vi "Pos2ndStrikerAfterPass.vi"(9 "AI Parameters":T1={"GotoKick"={"Dist do cone a frente"=150.0, "attacker farback"=1500.0, "Perto"=300.0, "min dist to kick"=150.0, "kick eps"=0.0, "Time to transition"=0.05}, "Attacker"={"CC chute"=0.09, "CC passe"=0.045, "Kick Force"=100.0, "ball-robot Kick"=200.0, "ball-robot Pass"=0.3, "drible\nAttk"=FALSE}, "Defender"={"D max"=1700.0, "Vel p/ robô av"=1000.0, "Kick Force"=100.0, "D atk-def"=0.0, "D farback"=0.0, "drible\ndef"=FALSE, "drible\ngoalie"=FALSE}, "Timeout"={"Field/v in x"=6.0, "Dist Robots"=300, "Dist up in y"=300}, "Pose Striker"={"dist"=200.0, "Numeric"=-4.0, "dist 2"=200.0, "drible\nstriker"=FALSE}, "Dist Stop"=300.0, "D ball out"=200, "D central gap "=150.0, "T pass"=0.0, "Force ++"=0.0, "range kick"=0.0, "Chute alto"=TRUE, "Marcador novo"=TRUE, "drible"=FALSE, "D drible"=300.0, "Versão Striker"=enum."3", "Defesa"=enum."ManMark", "Marcador"=enum."Marcar Segundo mais perigoso", "Receptor passe"=enum."2nd Striker", "Área"=enum."Quadrada"} {"D drible" format="%#_13g"; "D central gap" format="%#_13g"; "Dist Stop" format="%#_13g"; "Pose Striker"."Numeric" format="%#_13g"; "Defender"."Kick Force" format="%#_13g"; "Defender"."Vel p/ robô av" format="%#_13g"; "Attacker"."ball-robot Kick" format="%#_13g"; "Attacker"."Kick Force" format="%#_13g"; "Attacker"."CC passe" format="%#_13g"; "Attacker"."CC chute" format="%#_13g"; "GotoKick"."kick eps" format="%#_13g"; "GotoKick"."min dist to kick" format="%#_13g"; "GotoKick"."Perto" format="%#_13g"; "GotoKick"."attacker farback" format="%#_13g"; "GotoKick"."Dist do cone a frente" format="%#_13g"}, 10 "IA Input":T2={"our_robots"=[], "enemy_robots"=[], "balls"=[], "geometry"={"line_width"=0, "field_length"=0, "field_width"=0, "boundary_width"=0, "referee_width"=0, "goal_width"=0, "goal_depth"=0, "goal_wall_width"=0, "center_circle_radius"=0, "defense_radius"=0, "defense_stretch"=0, "free_kick_from_defense_dist"=0, "penalty_spot_from_field_line_dist"=0, "penalty_line_from_spot_dist"=0}, "IA Judge"={"stage"="", "command"="", "our_goalie_id"=0.0, "enemy_goalie_id"=0.0, "command enum"=enum."Halt", "Time"=enum."Azul"}, "Received Timestamp"=timestamp(0 s since 1904-01-01), "Events"={"Touch"=FALSE, "Ball out"=FALSE, "id touch"=0.0, "Ball out of \nVision"=FALSE, "Ball inside \nGoalie area"=FALSE, "Robot not responding"=FALSE, "Robots responding status"=[1.0, 1.0, 1.0, 1.0, 1.0, 1.0], "Enemy Ball \nPossession"=FALSE, "Pass State"=FALSE, "id end of pass"=0.0, "Kick"=FALSE, "Id ini Possession"=0.0, "Ball Possesion"=FALSE, "Id Possesion"=0.0, "Direct Kick"=FALSE, "2nd Strk Ativo"=FALSE}}, 11 "Robot in":T3={"id"=5, "function"=enum."Attacker", "x"=-1842.5054931640625, "y"=520.60986328125, "orientation"=-2.7555055618286133, "v_tangent"=0.0, "v_normal"=0.0, "v_ang"=0.0, "kick_x"=0.0, "kick_z"=0.0, "dribble"=FALSE, "Timestamp"=timestamp(2082758857.4639893 s since 1904-01-01), "estimatives"={"est_v_tangent"=0.0, "est_v_normal"=0.0, "est_vx"=0.0, "est_vy"=0.0, "Pos Robot Est"=[]}, "dest_x_kick"=0.0, "dest_y_kick"=0.0, "Gap Coord"=[], "States"=enum."GoToTangent", "Path "=[], "Path  Smooth"=[], "Dest"=[]}) -> (3 "Robot out":T3={"id"=5, "function"=enum."Attacker", "x"=-1842.5054931640625, "y"=520.60986328125, "orientation"=-2.7555055618286133, "v_tangent"=-0.08361641967936218, "v_normal"=-0.20513016702014014, "v_ang"=0.24456003022714357, "kick_x"=0.0, "kick_z"=0.0, "dribble"=FALSE, "Timestamp"=timestamp(2082758857.4639893 s since 1904-01-01), "estimatives"={"est_v_tangent"=0.0, "est_v_normal"=0.0, "est_vx"=0.0, "est_vy"=0.0, "Pos Robot Est"=[]}, "dest_x_kick"=0.0, "dest_y_kick"=0.0, "Gap Coord"=[], "States"=enum."GoToTangent", "Path "=[], "Path  Smooth"=[], "Dest"=[]})   [LabVIEW 2017]
uses:
  Core/AI Robot.ctl
  Functions Enum.ctl
  AttackerStates.ctl
  Path Planning/RRT/PathDests.ctl
  Path Planning/RRT/PathDest.ctl
  Core/AI Input.ctl
  Core/AI Ball.ctl
  Core/Field Size.ctl
  Core/AI Judge.ctl
  Command Enum.ctl
  Util/Events/Events.ctl
  AI Parameters.ctl
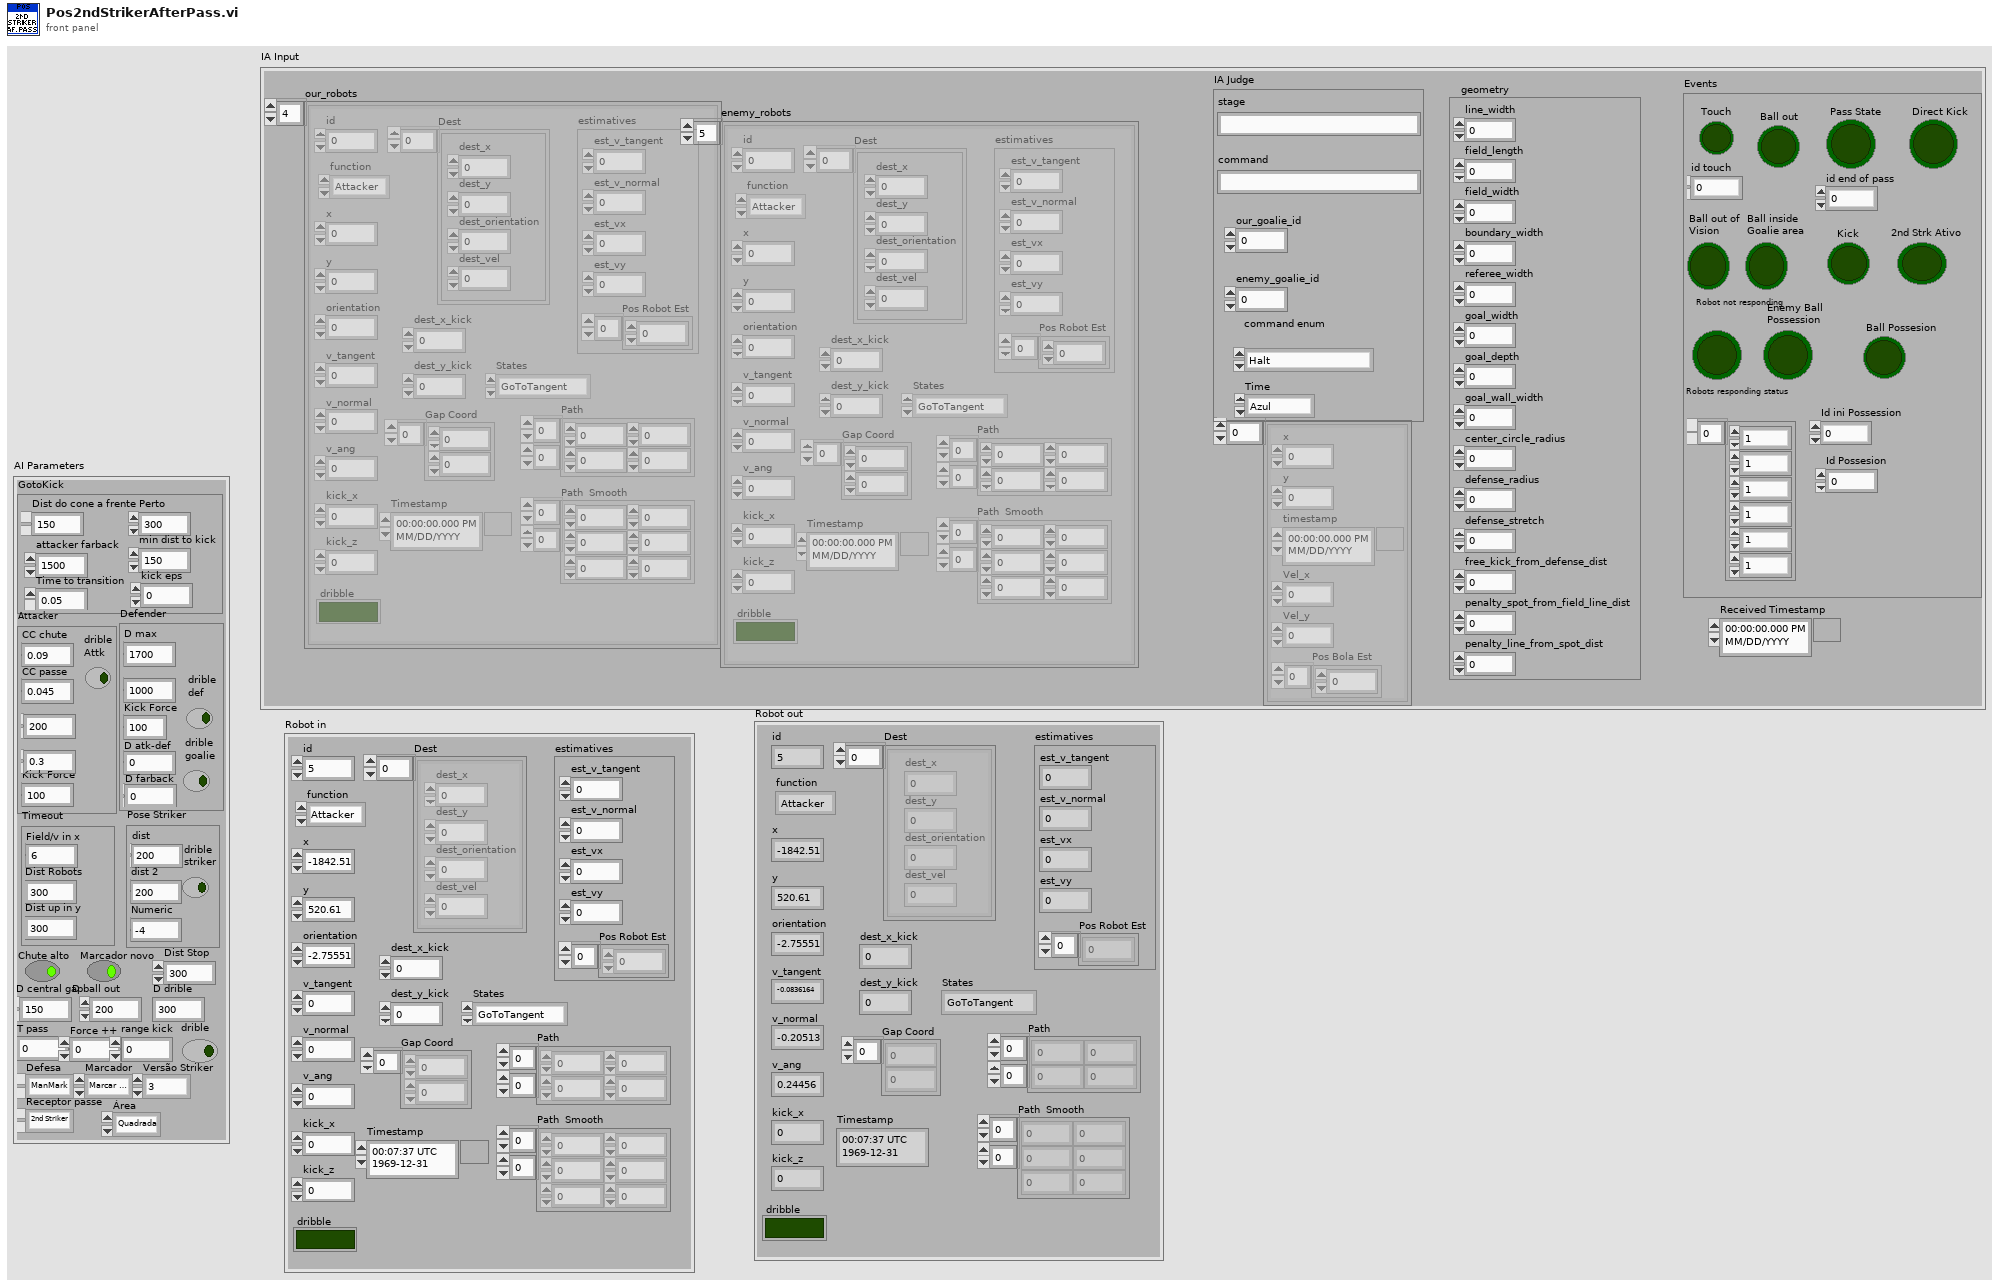
[diagram p1: front panel]
types:
  T1 = typedef "AI Parameters.ctl" = cluster{"GotoKick":cluster{"Dist do cone a frente":dbl, "attacker farback":dbl, "Perto":dbl, "min dist to kick":dbl, "kick eps":dbl, "Time to transition":dbl}, "Attacker":cluster{"CC chute":dbl, "CC passe":dbl, "Kick Force":dbl, "ball-robot Kick":dbl, "ball-robot Pass":dbl, "drible\nAttk":bool}, "Defender":cluster{"D max":dbl, "Vel p/ robô av":dbl, "Kick Force":dbl, "D atk-def":dbl, "D farback":dbl, "drible\ndef":bool, "drible\ngoalie":bool}, "Timeout":cluster{"Field/v in x":dbl, "Dist Robots":u32, "Dist up in y":u32}, "Pose Striker":cluster{"dist":dbl, "Numeric":dbl, "dist 2":dbl, "drible\nstriker":bool}, "Dist Stop":dbl, "D ball out":i32, "D central gap ":dbl, "T pass":dbl, "Force ++":dbl, "range kick":dbl, "Chute alto":bool, "Marcador novo":bool, "drible":bool, "D drible":dbl, "Versão Striker":enum16{"Auto", "3", "2", "1"}, "Defesa":enum16{"ManMark", "Barreira"}, "Marcador":enum16{"Marcar Segundo mais perigoso", "Marcar o mais perigoso"}, "Receptor passe":enum16{"Auto", "2nd Striker", "Striker"}, "Área":enum16{"Quadrada", "Circular"}}
  T2 = typedef "AI Input.ctl" = cluster{"our_robots":T3[], "enemy_robots":T3[], "balls":T8[], "geometry":T9, "IA Judge":T10, "Received Timestamp":timestamp, "Events":T12}
  T3 = typedef "AI Robot.ctl" = cluster{"id":u32, "function":T4, "x":dbl, "y":dbl, "orientation":dbl, "v_tangent":dbl, "v_normal":dbl, "v_ang":dbl, "kick_x":dbl, "kick_z":dbl, "dribble":bool, "Timestamp":timestamp, "estimatives":cluster{"est_v_tangent":dbl, "est_v_normal":dbl, "est_vx":dbl, "est_vy":dbl, "Pos Robot Est":dbl[]}, "dest_x_kick":dbl, "dest_y_kick":dbl, "Gap Coord":dbl[], "States":T5, "Path ":dbl[][], "Path  Smooth":dbl[][], "Dest":T6}
  T4 = typedef "Functions Enum.ctl" = enum16{"2nd Striker", "Attacker", "Goalie", "Defender", "Striker", "Goto 0", "Dummy", "Kicker", "ZigZag 0", "ZigZag 1", "ZigZag 2", "ZigZag 3", "ZigZag 4", "ZigZag 5", "ZigZag 6", "ZigZag 7", "ZigZag 8", ""}
  T5 = typedef "AttackerStates.ctl" = enum16{"Pass", "GoToTangent", "BallGetting", "GoToKick", ""}
  T6 = typedef "PathDests.ctl" = T7[]
  T7 = typedef "PathDest.ctl" = cluster{"dest_x":dbl, "dest_y":dbl, "dest_orientation":dbl, "dest_vel":dbl}
  T8 = typedef "AI Ball.ctl" = cluster{"x":dbl, "y":dbl, "timestamp":timestamp, "Vel_x":dbl, "Vel_y":dbl, "Pos Bola Est":dbl[]}
  T9 = typedef "Field Size.ctl" = cluster{"line_width":u32, "field_length":u32, "field_width":u32, "boundary_width":u32, "referee_width":u32, "goal_width":u32, "goal_depth":u32, "goal_wall_width":u32, "center_circle_radius":u32, "defense_radius":u32, "defense_stretch":u32, "free_kick_from_defense_dist":u32, "penalty_spot_from_field_line_dist":u32, "penalty_line_from_spot_dist":u32}
  T10 = typedef "AI Judge.ctl" = cluster{"stage":string, "command":string, "our_goalie_id":dbl, "enemy_goalie_id":dbl, "command enum":T11, "Time":enum16{"Azul", "Amarelo"}}
  T11 = typedef "Command Enum.ctl" = enum16{"Halt", "Stop", "Force Start", "PKA Normal Start", "Prepare Kickoff Ally", "PKE Normal Start", "Prepare Kickoff Enemy", "Prepare Penalty Ally", "PPA Normal Start", "Prepare Penalty Enemy", "PPE Normal Start", "Direct Free Enemy", "Direct Free Ally", "Indirect Free Enemy", "Indirect Free Ally", "Timeout Enemy", "Timeout Ally", "Goal Enemy", "Goal Ally", "Ball Placement Enemy", "Ball Placement Ally", "Normal Half Time", "Extra Time Break", "Extra Half Time", "None", "Post Game"}
  T12 = typedef "Events.ctl" = cluster{"Touch":bool, "Ball out":bool, "id touch":dbl, "Ball out of \nVision":bool, "Ball inside \nGoalie area":bool, "Robot not responding":bool, "Robots responding status":dbl[], "Enemy Ball \nPossession":bool, "Pass State":bool, "id end of pass":dbl, "Kick":bool, "Id ini Possession":dbl, "Ball Possesion":bool, "Id Possesion":dbl, "Direct Kick":bool, "2nd Strk Ativo":bool}
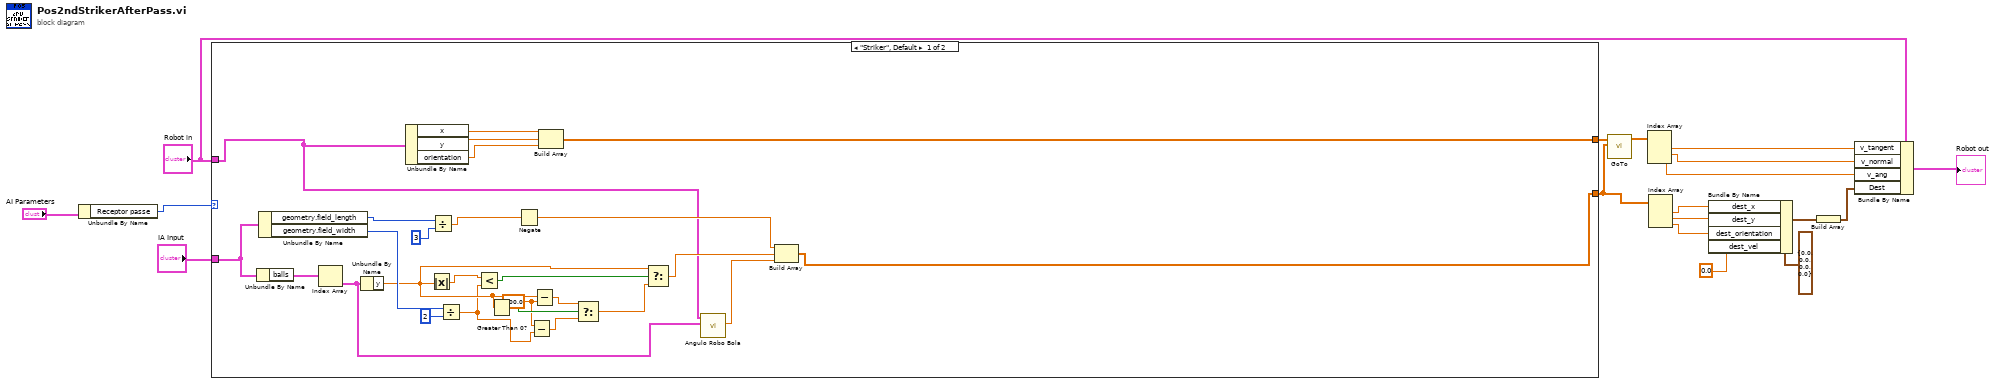
[diagram p0: block diagram]
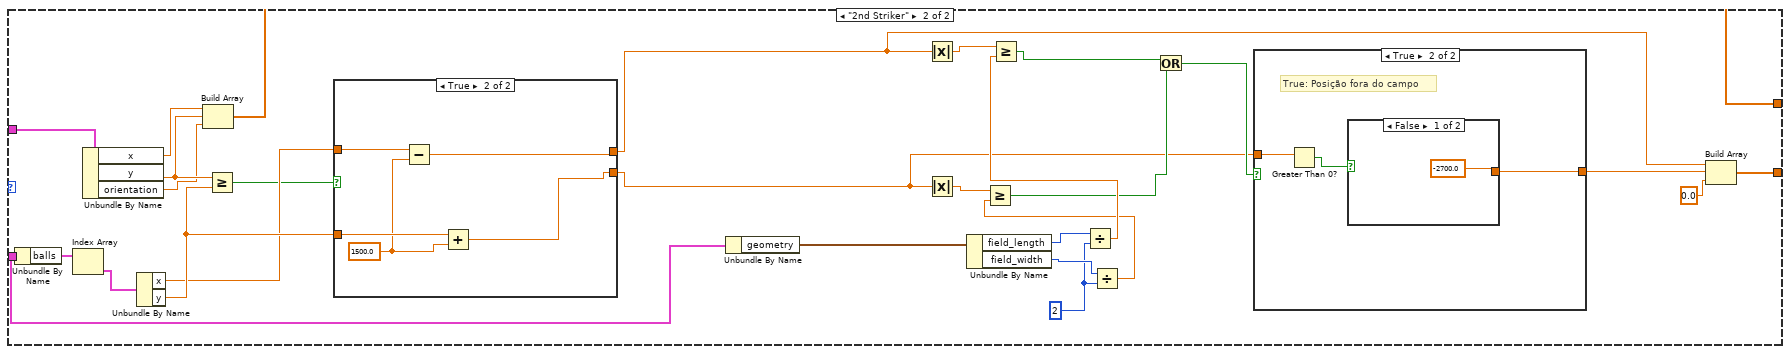
[diagram p2: hidden frame]
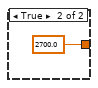
[diagram p4: hidden frame]
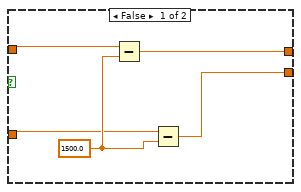
[diagram p5: hidden frame]
diagram:
  n1 = Unbundle By Name("AI Parameters") -> ("Receptor passe"=w1:enum16{"Auto", "2nd Striker", "Striker"})
  n2 = case shown="\"Striker\", Default" w1 {
    tunnel: "Robot in" -> [w21 w66]
    tunnel: [w19 w64] -> w5
    tunnel: "IA Input" -> [w22 w56]
    tunnel: [w20 w45] -> w3
    frame "Striker", Default {
      w33 = 300.0 ("y")
      n3 = Unbundle By Name(w22) -> ("balls"=w42:T8[])
      n4 = Unbundle By Name(w22) -> ("geometry.field_length"=w44:u32, "geometry.field_width"=w40:u32)
      n5 = Index Array(array=w42) -> (element=w29:T8)  [unwired: 1 in]
      n6 = Unbundle By Name(w29) -> ("y"=w35:dbl)
      n7 = Unbundle By Name(w21) -> ("x"=w27:dbl, "y"=w26:dbl, "orientation"=w25:dbl)
      n8 = Absolute Value(x=w35) -> (abs(x)=w41:dbl)
      n9 = Divide(x=w44, y=u32 3) -> (x/y=w24:dbl)
      n10 = Divide(x=w40, y=u32 2) -> (x/y=w32:dbl)
      n11 = Less?(x=w41, y=w32) -> (x < y?=w38:bool)
      n12 = Greater Than 0?(x=w35) -> (x > 0?=w37:bool)
      n13 = Negate(x=w24) -> (-x=w23:dbl)
      n14 = Subtract(x=w33, y=w32) -> (x-y=w31:dbl)
      n15 = Subtract(x=w35, y=w33) -> (x-y=w34:dbl)
      n16 = Build Array(w27, w26, w25) -> (w20:dbl[])
      n17 = Select(t=w34, s=w37, f=w31) -> (s? t:f=w36:dbl)
      n18 = Select(t=w35, s=w38, f=w36) -> (s? t:f=w30:dbl)
      n19 = call "Angulo Robo Bola.vi"("Ball"=w29, "Robot"=w21) -> ("Angulo"=w28:dbl)  [unwired: 9 in]
      n20 = Build Array(w23, w30, w28) -> (w19:dbl[])
    }
    frame "2nd Striker" {
      w49 = u32 2 ("field_length")
      n21 = Unbundle By Name(w56) -> ("balls"=w71:T8[])
      n22 = Index Array(array=w71) -> (element=w70:T8)  [unwired: 1 in]
      n23 = Unbundle By Name(w66) -> ("x"=w48:dbl, "y"=w47:dbl, "orientation"=w46:dbl)
      n24 = Unbundle By Name(w70) -> ("x"=w68:dbl, "y"=w69:dbl)
      n25 = Build Array(w48, w47, w46) -> (w45:dbl[])
      n26 = Greater Or Equal?(x=w47, y=w69) -> (x >= y?=w67:bool)
      n27 = case shown="True" w67 {
        tunnel: w69 -> [w81 w87]
        tunnel: w68 -> [w80 w86]
        tunnel: [w79 w84] -> w50
        tunnel: [w78 w83] -> w52
        frame False {
          w82 = 1500.0 ("y")
          n28 = Subtract(x=w80, y=w82) -> (x-y=w79:dbl)
          n29 = Subtract(x=w81, y=w82) -> (x-y=w78:dbl)
        }
        frame True {
          w85 = 1500.0 ("y")
          n30 = Subtract(x=w86, y=w85) -> (x-y=w84:dbl)
          n31 = Add(x=w87, y=w85) -> (x+y=w83:dbl)
        }
      }
      n32 = Unbundle By Name(w56) -> ("geometry"=w63:T9)
      n33 = Absolute Value(x=w50) -> (abs(x)=w54:dbl)
      n34 = Absolute Value(x=w52) -> (abs(x)=w59:dbl)
      n35 = Unbundle By Name(w63) -> ("field_length"=w62:u32, "field_width"=w61:u32)
      n36 = Divide(x=w62, y=w49) -> (x/y=w60:dbl)
      n37 = Greater Or Equal?(x=w54, y=w60) -> (x >= y?=w55:bool)
      n38 = Divide(x=w61, y=w49) -> (x/y=w58:dbl)
      n39 = Greater Or Equal?(x=w59, y=w58) -> (x >= y?=w57:bool)
      n40 = Or(x=w55, y=w57) -> (x .or. y?=w53:bool)
      n41 = case shown="True" w53 {
        tunnel: w52 -> [w72 w75]
        tunnel: [w72 w73] -> w51
        frame False {
          # "True: Posição detnro do campo"
        }
        frame True {
          # "True: Posição fora do campo"
          n42 = Greater Than 0?(x=w75) -> (x > 0?=w74:bool)
          n43 = case shown="False" w74 {
            tunnel: [-2700.0 2700.0] -> w73
            frame False {
            }
            frame True {
            }
          }
        }
      }
      n44 = Build Array(w50, w51, 0.0 ("element")) -> (w64:dbl[])
    }
  }
  n45 = call "GoTo.vi"("Target"=w5, "Position"=w3) -> ("Output\nVelocity"=w18:dbl[])  [unwired: 8 in, 1 out]
  n46 = Index Array(array=w18) -> (element #1=w17:dbl, element #2=w16:dbl, element #3=w15:dbl)  [unwired: 3 in]
  n47 = Index Array(array=w5) -> (element #1=w10:dbl, element #2=w9:dbl, element #3=w8:dbl)  [unwired: 3 in]
  n48 = Bundle By Name(cluster=T7 {"dest_x"=0.0, "dest_y"=0.0, "dest_orientation"=0.0, "dest_vel"=0.0} ("Dest"), "dest_x"=w10, "dest_y"=w9, "dest_orientation"=w8, "dest_vel"=0.0) -> (w13:T7)
  n49 = Build Array(w13) -> (w11:T7[])
  n50 = Bundle By Name(cluster="Robot in", "v_tangent"=w17, "v_normal"=w16, "v_ang"=w15, "Dest"=w11) -> (→"Robot out":T3)
